vi "Set Target.vi"(7 "error in":errorcluster, 8 "Target":i16, 9 "Actuator name":string, 10 "UTP IO Session in":T1) -> (0 "error out":errorcluster, 2 "Actuator was Ready?":bool=TRUE, 3 "UTP IO Session out":T1)   [LabVIEW 2023, in "Actuators.lvlib"]
doc: "Target 100 - Home position\nTarget 101 - Work position\nExpiredTimeToWait? => Rising/Falling edge wasn't detected\nThis VI will perform actuator action, if actutor is Ready (No errors)\nReading period is 10ms"
uses:
  Actuators.lvlib
  <vilib>/Noffz/UTP IO/UTP IO Library/Typedefs/Session Handle.ctl
  <vilib>/Noffz/UTP IO/UTP IO Library/UTP IO Pool Session.lvclass
  <vilib>/Noffz/UTP IO/UTP IO Library/methods/poly/plc/Write PLC Variable (I16).vi
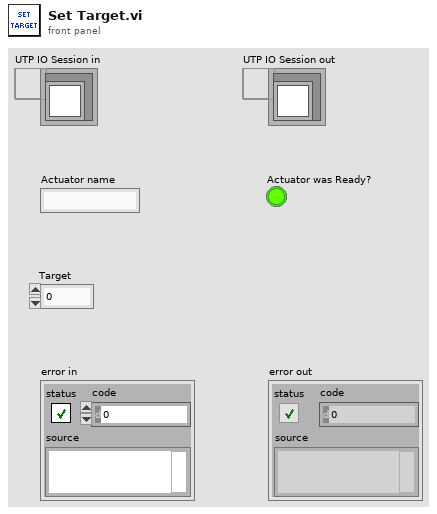
[diagram p1: front panel]
types:
  T1 = typedef "UTP IO Library.lvlib/UTP IO Pool Session.lvclass/Session Handle.ctl" = refnum<data-value>
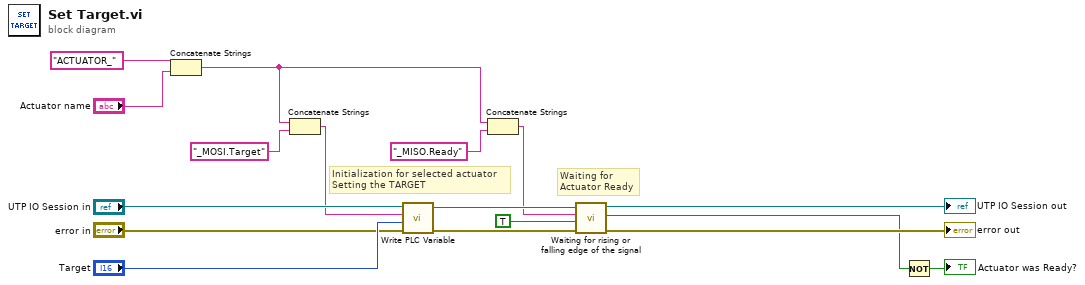
[diagram p0: block diagram]
diagram:
  # "Waiting for \nActuator Ready"
  # "Initialization for selected actuator\nSetting the TARGET"
  n1 = Concatenate Strings("ACTUATOR_" ("string"), "Actuator name") -> (w9:string)
  n2 = Concatenate Strings(w9, "_MOSI.Target" ("string")) -> (w14:string)
  n3 = call-poly <vilib>:"Write PLC Variable.vi"("error in (no error)"="error in", "value"="Target", "variable name"=w14, "UTP IO Session in"="UTP IO Session in") -> ("error out"=w13:errorcluster, "UTP IO Session out"=w16:T1)  [unwired: 6 in]
  n4 = Concatenate Strings(w9, "_MISO.Ready" ("string")) -> (w7:string)
  n5 = call "Waiting for rising or falling edge of the signal.vi"("error in"=w13, "Rising/Falling edge"=TRUE, "Variable name"=w7, "UTP IO Session in"=w16) -> ("error out"=→"error out":errorcluster, "ExpiredTimeToWait?"=w1:bool, "UTP IO Session out"=→"UTP IO Session out":T1)  [unwired: 5 in]
  n6 = Not(x=w1) -> (.not. x?=→"Actuator was Ready?":bool)
